vi "Act.vi"(8 "error in (no error)":errorcluster, 9 "VI Refnum in":refnum<vi>, 10 "Flex Msg type":refnum<class "Flex Msg.lvclass">, 11 "Data Access Handler in":refnum<class "Data Access Handler.lvclass">) -> (0 "error out":errorcluster, 1 "Await user action?":bool, 3 "Data Access Handler out":refnum<class "Data Access Handler.lvclass">)   [LabVIEW 2020, in "Msg.lvlib" / "Data Access Handler.lvclass"]
doc: "Default implementation does nothing."
uses:
  Data Access Handler.lvclass
  Flex Msg.lvclass
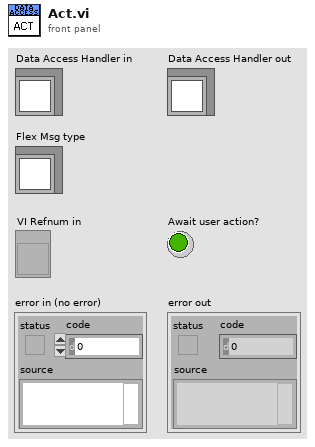
[diagram p1: front panel]
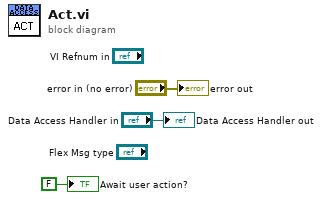
[diagram p0: block diagram]
diagram:
  "error out" <- "error in (no error)"
  "Data Access Handler out" <- "Data Access Handler in"
  "Await user action?" <- FALSE ("Await user action?")
